vi "Num Count Step Sign.vi"(9 "Step Size In":dbl=0.1 min=0.1, 10 "Stop value":dbl, 11 "Start Value":dbl) -> (2 "Step size out":dbl, 3 "Number":dbl)   [LabVIEW 2024]
doc: "This VI takes three inputs , Start, Stop, and Step size to calculate the number of measurements to be done. This also assign the proper sign of step size. If Start value is greater than Stop value, then it automatically changes the step size to negative, so that the next setpoint can be found by just adding the step size into start value."
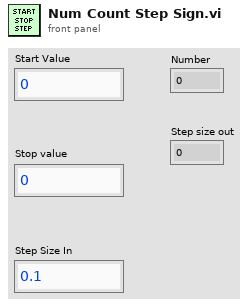
[diagram p1: front panel]
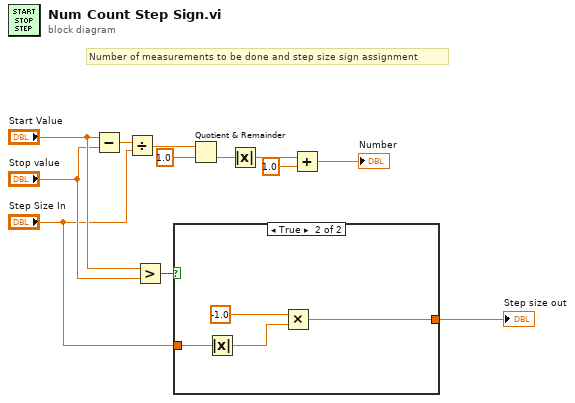
[diagram p0: block diagram]
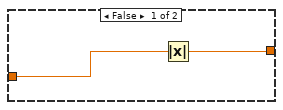
[diagram p2: hidden frame]
diagram:
  # "Number of measurements to be done and step size sign assignment"
  n1 = Subtract(x="Start Value", y="Stop value") -> (x-y=w6:dbl)
  n2 = Divide(x=w6, y="Step Size In") -> (x/y=w7:dbl)
  n3 = Greater?(x="Start Value", y="Stop value") -> (0:w5:bool)
  n4 = case shown="True" w5 {
    tunnel: "Step Size In" -> [w13 w16]
    tunnel: [w14 w15] -> w1
    frame False {
      n5 = Absolute Value(x=w13) -> (abs(x)=w14:dbl)
    }
    frame True {
      n6 = Absolute Value(x=w16) -> (abs(x)=w17:dbl)
      n7 = Multiply(x=-1.0, y=w17) -> (x*y=w15:dbl)
    }
  }
  "Step size out" <- w1
  n8 = Quotient & Remainder(x=w7, y=1.0) -> (floor(x/y)=w8:dbl)  [unwired: 1 out]
  n9 = Absolute Value(x=w8) -> (abs(x)=w9:dbl)
  n10 = Add(x=w9, y=1.0) -> (x+y=→"Number":dbl)
